vi "RT-Weight-Order.vi"() -> ()   [LabVIEW 2020]
panel:
  out "Array3":dbl[](array[numeric])
  out "Array 2":dbl[](array[numeric])
  out "Array1":dbl[](array[numeric])
  out "Array 0":dbl[](array[numeric])
  out "Weights":T1
  in  "Input":string[][](array[string])
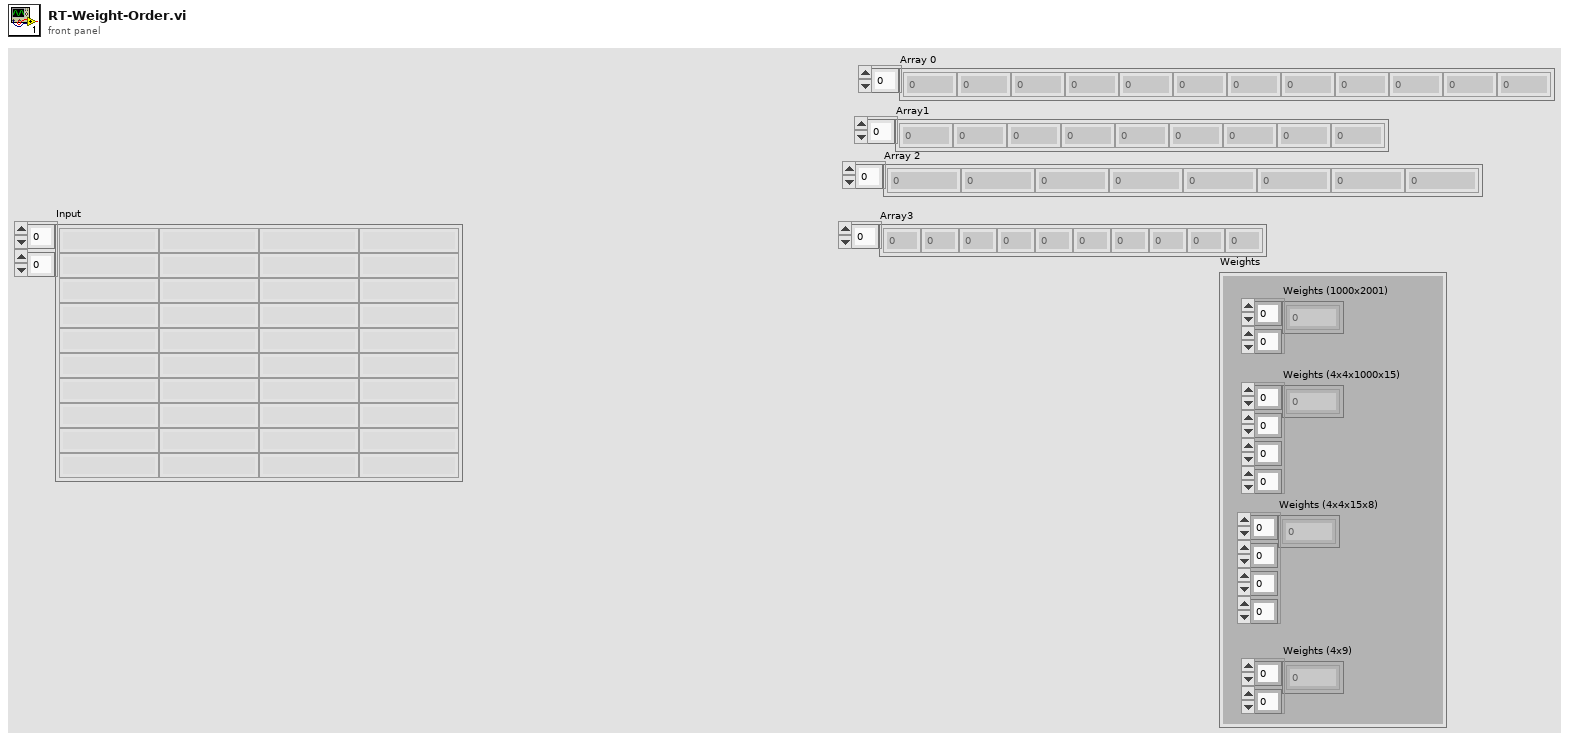
[diagram p1: front panel]
types:
  T1 = cluster{"Weights (1000x2001)":dbl[][], "Weights (4x4x1000x15)":dbl[][][][], "Weights (4x4x15x8)":dbl[][][][], "Weights (4x9)":dbl[][]}
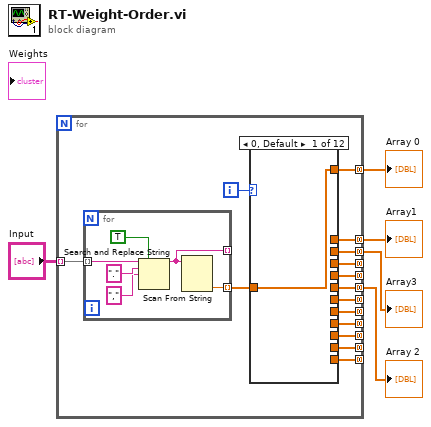
[diagram p0: block diagram]
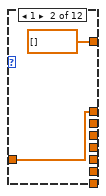
[diagram p2: hidden frame]
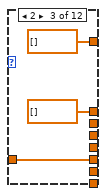
[diagram p3: hidden frame]
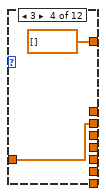
[diagram p4: hidden frame]
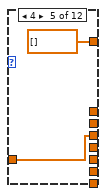
[diagram p5: hidden frame]
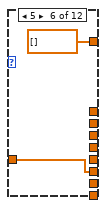
[diagram p6: hidden frame]
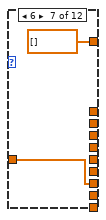
[diagram p7: hidden frame]
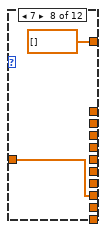
[diagram p8: hidden frame]
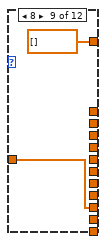
[diagram p9: hidden frame]
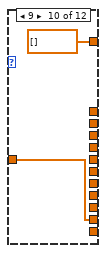
[diagram p10: hidden frame]
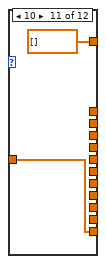
[diagram p11: hidden frame]
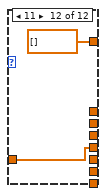
[diagram p12: hidden frame]
diagram:
  n1 = for {
    tunnel: "Input" -> [w20] mode=indexing
    tunnel: [w18] -> w4 mode=concatenating
    tunnel: [w17] -> w3 mode=concatenating
    tunnel: [w16] -> w2 mode=concatenating
    tunnel: [w15] -> w1 mode=concatenating
    tunnel: [w14] -> _ mode=concatenating
    tunnel: [w13] -> _ mode=concatenating
    tunnel: [w12] -> _ mode=concatenating
    tunnel: [w11] -> _ mode=concatenating
    tunnel: [w10] -> _ mode=concatenating
    tunnel: [w9] -> _ mode=concatenating
    tunnel: [w8] -> _ mode=concatenating
    tunnel: [w7] -> _ mode=concatenating
    i -> [w19]
    n2 = for {
      tunnel: w20 -> [w50] mode=indexing
      tunnel: [w46] -> _ mode=indexing
      tunnel: [w45] -> w6 mode=indexing
      n3 = Search and Replace String(replace all?=TRUE ("replace all? (F)"), input string=w50, search string=".", replace string="," ("replace string (\"\")")) -> (result string=w46:string)  [unwired: 4 in, 3 out]
      n4 = Scan From String(input string=w46) -> (output 1=w45:dbl)  [unwired: 4 in, 3 out]
    }
    n5 = case shown="0, Default" w19 {
      tunnel: w6 -> [w21 w23 w24 w28 w29 w31 w33 w35 w37 w39 w41 w43]
      tunnel: [w21 dbl[] [] dbl[] [] dbl[] [] dbl[] [] dbl[] [] dbl[] [] dbl[] [] dbl[] [] dbl[] [] dbl[] [] dbl[] []] -> w18
      tunnel: [_ w23 dbl[] [] _ _ _ _ _ _ _ _ _] -> w17
      tunnel: [_ _ w24 _ _ _ _ _ _ _ _ _] -> w16
      tunnel: [_ _ _ w28 _ _ _ _ _ _ _ _] -> w15
      tunnel: [_ _ _ _ w29 _ _ _ _ _ _ _] -> w14
      tunnel: [_ _ _ _ _ w31 _ _ _ _ _ _] -> w13
      tunnel: [_ _ _ _ _ _ w33 _ _ _ _ _] -> w12
      tunnel: [_ _ _ _ _ _ _ w35 _ _ _ _] -> w11
      tunnel: [_ _ _ _ _ _ _ _ w37 _ _ _] -> w10
      tunnel: [_ _ _ _ _ _ _ _ _ w39 _ _] -> w9
      tunnel: [_ _ _ _ _ _ _ _ _ _ w41 _] -> w8
      tunnel: [_ _ _ _ _ _ _ _ _ _ _ w43] -> w7
      frame 0, Default {
      }
      frame 1 {
      }
      frame 2 {
      }
      frame 3 {
      }
      frame 4 {
      }
      frame 5 {
      }
      frame 6 {
      }
      frame 7 {
      }
      frame 8 {
      }
      frame 9 {
      }
      frame 10 {
      }
      frame 11 {
      }
    }
  }
  "Array 0" <- w4
  "Array1" <- w3
  "Array 2" <- w2
  "Array3" <- w1
